vi "xControlTest.vi"() -> ()   [LabVIEW 2012]
uses:
  Time Slider.xctl
panel:
  in  "Time Slider 2":cluster{"Data":dbl, "Data 2":dbl, "Data 3":dbl}(xcontrol)
  in  "stop":bool
  in  "Min":dbl
  in  "Max":dbl
  in  "Time Slider":cluster{"Data":dbl, "Data 2":dbl, "Data 3":dbl}(xcontrol)
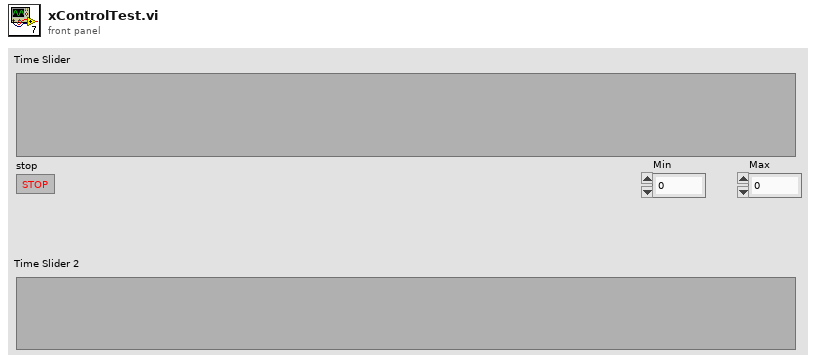
[diagram p1: front panel]
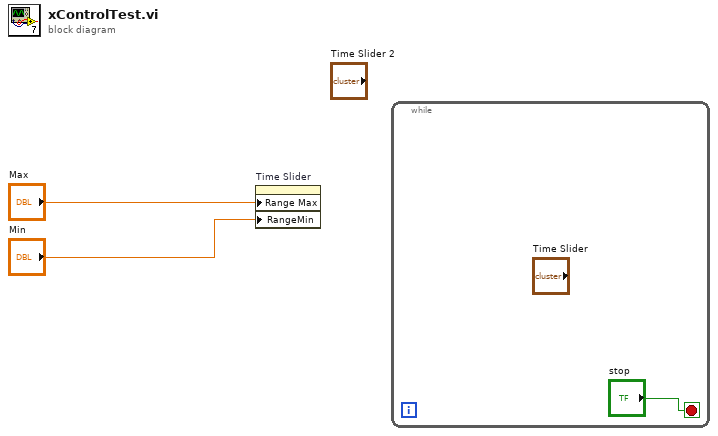
[diagram p0: block diagram]
diagram:
  n1 = property on="Time Slider" class="Time Slider (strict)"("Range Max"="Max", "RangeMin"="Min") -> ()  [unwired: 2 in, 2 out]
  n2 = while {
    stop <- "stop" stop-if-true
  }
